vi "writeSingleCommand.vi"(4 "String":string, 8 "error out":errorcluster, 9 "Session Hash":u64, 10 "NetworkStreamCluster":T2, 11 "endpoint input":refnum<k21>) -> (0 "error IO":errorcluster, 2 "next move":T1)   [LabVIEW 2018]
uses:
  NetworkStream/NetworkStreamData.ctl
  Tektronik3102/Tecktronik action loop.ctl
  NetworkStream/NetworkStream.lvlib
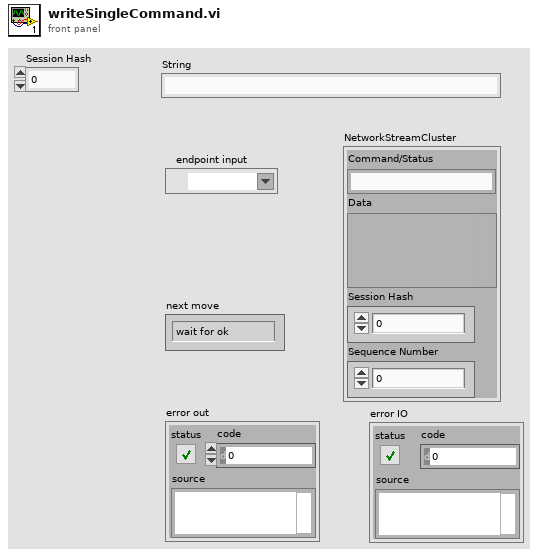
[diagram p1: front panel]
types:
  T1 = typedef "Tecktronik action loop.ctl" = enum16{"wait for ok", "error", "ready", "write log file", "waiting for connection", "exit", "sending command"}
  T2 = typedef "NetworkStream.lvlib/NetworkStreamData.ctl" = cluster{"Command/Status":string, "Data":variant, "Session Hash":u64, "Sequence Number":u64}
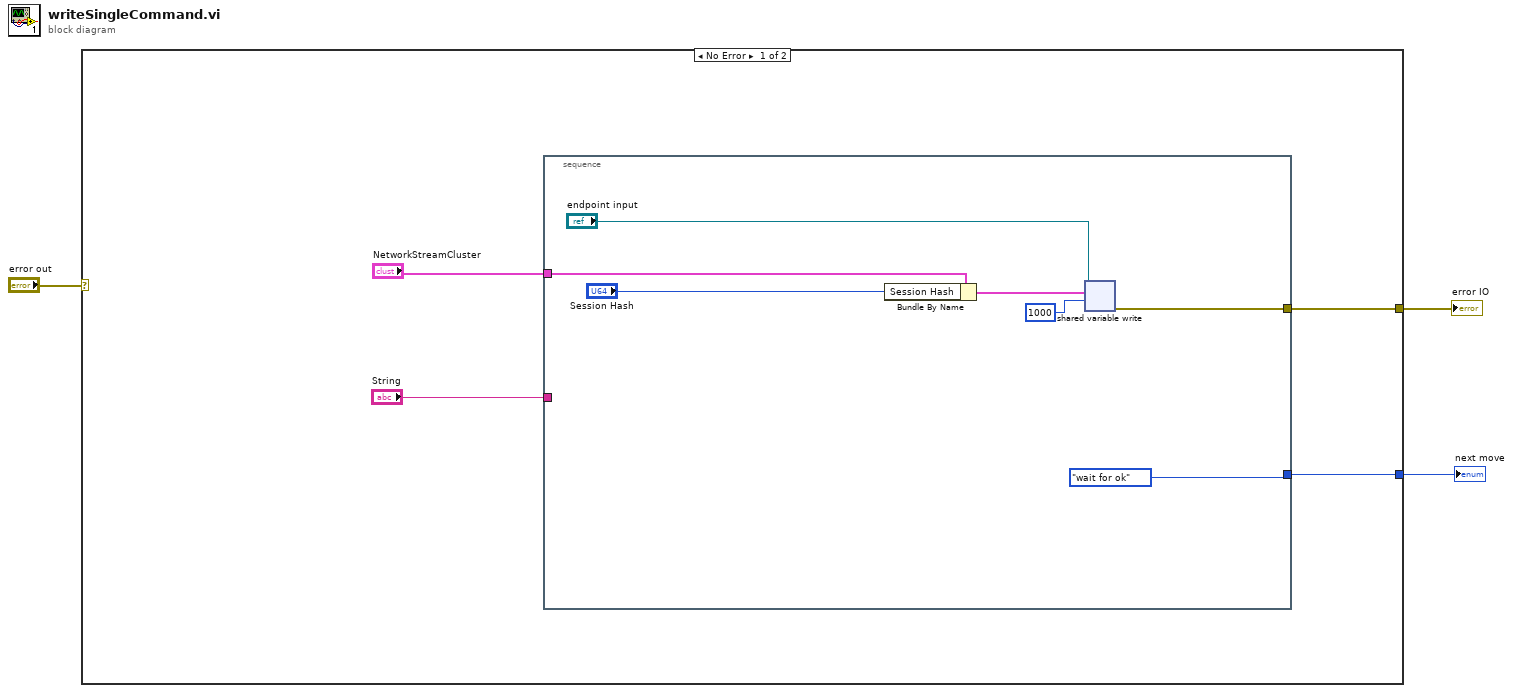
[diagram p0: block diagram]
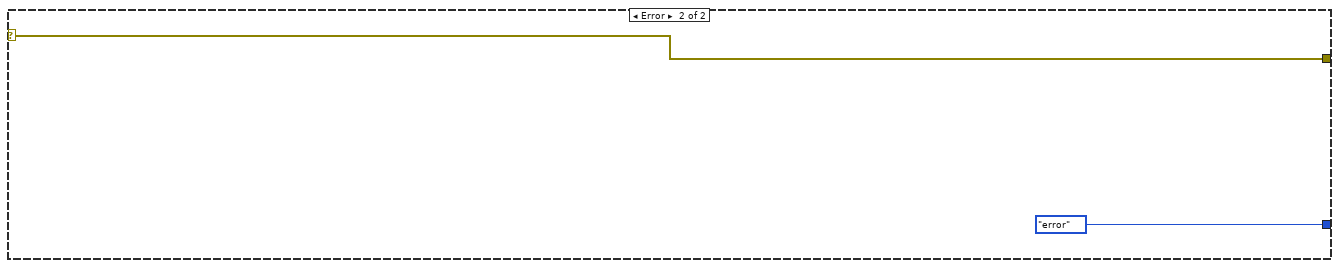
[diagram p2: hidden frame]
diagram:
  n1 = case shown="No Error" "error out" {
    selector: "error out" -> [_ w16]
    tunnel: [w7 w16] -> w2
    tunnel: [w6 Tecktronik_action_loop."error" ("next move")] -> w1
    frame No Error {
      n2 = stacked-sequence {
        tunnel: [w13] -> w7
        tunnel: [Tecktronik_action_loop."wait for ok" ("next move")] -> w6
        tunnel: "NetworkStreamCluster" -> [w9]
        tunnel: "String" -> [_]
        frame #0 {
          n3 = Bundle By Name(cluster=w9, "Session Hash"="Session Hash") -> (w12:T2)
          n4 = shared-variable-write ("Write Single Element to Stream")("endpoint input", w12, 1000 ("timeout ms (-1)")) -> (w13:errorcluster)  [unwired: 1 in, 2 out]
        }
      }
    }
    frame Error {
    }
  }
  "error IO" <- w2
  "next move" <- w1
